vi "close connection.vi"(8 "error in":errorcluster, 11 "Serial Master in":refnum<class "Serial Data Unit.lvclass">) -> (0 "error out":errorcluster, 3 "Serial Master out":refnum<class "Serial Data Unit.lvclass">)   [LabVIEW 2021, in "Serial Data Unit.lvclass"]
doc: "This provides an interface for the master to close a connection to the slave."
uses:
  Serial Data Unit.lvclass
  Serial Data Unit.lvclass/Serial Data Unit.ctl
  Read visa resource name.vi
  Write visa resource name.vi
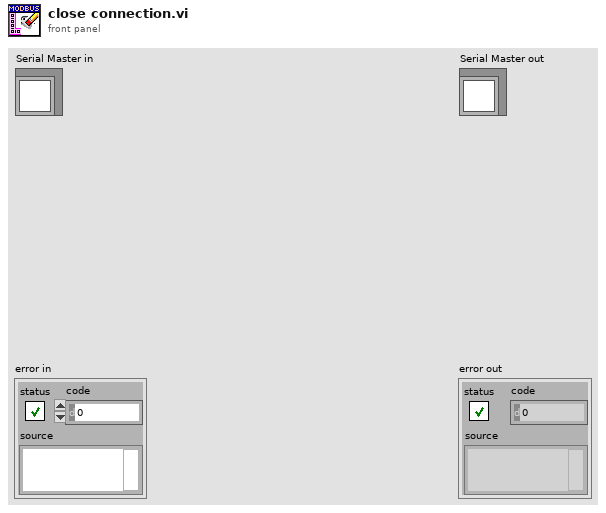
[diagram p1: front panel]
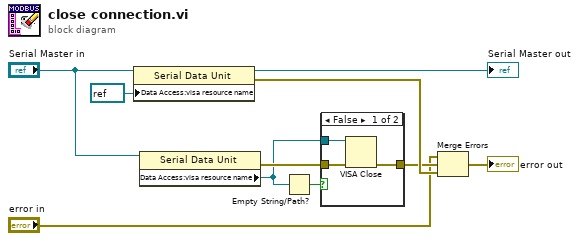
[diagram p0: block diagram]
diagram:
  n1 = property class="Serial Data Unit"(reference="Serial Master in", "Data Access:visa resource name"=refnum<visa-resource-name> refnum ("VISA resource name")) -> (reference out=→"Serial Master out":refnum<class "Serial Data Unit.lvclass">, error out=w6:errorcluster)  [unwired: 1 in]
  n2 = property class="Serial Data Unit"(reference="Serial Master in") -> (error out=w10:errorcluster, "Data Access:visa resource name"=w9:refnum<visa-resource-name>)  [unwired: 1 in, 1 out]
  n3 = Empty String/Path?(string/path=w9) -> (empty?=w8:bool)
  n4 = case shown="False" w8 {
    tunnel: w10 -> [w13 w14]
    tunnel: [w12 w14] -> w5
    tunnel: w9 -> [w11 _]
    frame False {
      n5 = VISA Close(VISA resource name=w11, error in (no error)=w13) -> (error out=w12:errorcluster)
    }
    frame True {
    }
  }
  n6 = Merge Errors("error in", w5, w6) -> (→"error out":errorcluster)
